vi "Thread Loop.vi"(8 "error in (no error)":errorcluster, 11 "Thread in":refnum<class "Thread.lvclass">) -> (0 "error out":errorcluster, 3 "Thread out":refnum<class "Thread.lvclass">)   [LabVIEW 2012, in "Architecture.lvlib" / "Thread.lvclass"]
uses:
  Thread.lvclass
  Message/Message.lvclass
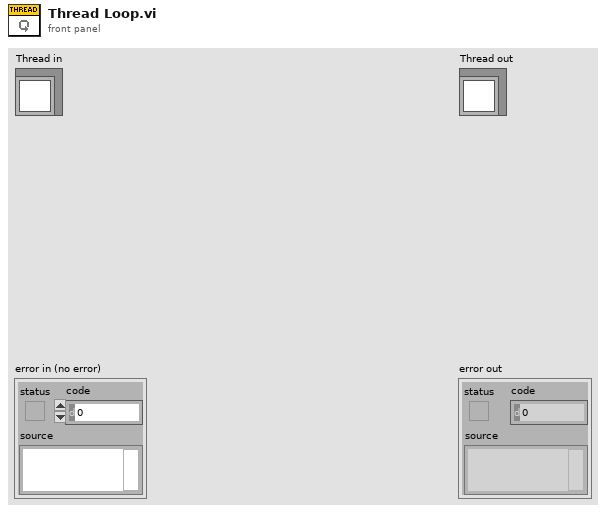
[diagram p1: front panel]
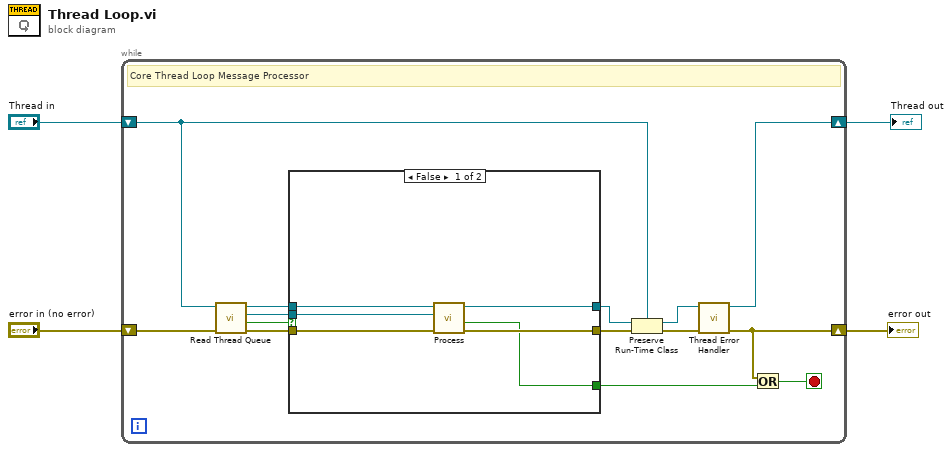
[diagram p0: block diagram]
diagram:
  n1 = while {
    shift-right: [w9] -> w1
    shift-left: "Thread in" -> [w13]
    shift-right: [w7] -> w2
    shift-left: "error in (no error)" -> [w18]
    stop <- w6 stop-if-true
    # "Core Thread Loop Message Processor"
    n2 = call "Read Thread Queue.vi"("error in (no error)"=w18, "Thread in"=w13) -> ("error out"=w16:errorcluster, "timed out?"=w17:bool, "Message"=w8:refnum<class "Message.lvclass">, "Thread out"=w15:refnum<class "Thread.lvclass">)  [unwired: 6 in]
    n3 = case shown="False" w17 {
      tunnel: w16 -> [w24 w25]
      tunnel: [w23 w25] -> w14
      tunnel: w15 -> [w22 w26]
      tunnel: [w21 w26] -> w12
      tunnel: w8 -> [w20 _]
      tunnel: [w19 _] -> w5
      frame False {
        n4 = call-dynamic "Process.vi"("error in (no error)"=w24, "Message in"=w20, "Architecture.lvlib:Thread.lvclass"=w22) -> ("error out"=w23:errorcluster, "Stop?"=w19:bool, "Architecture.lvlib:Thread.lvclass 2"=w21:refnum<class "Thread.lvclass">)  [unwired: 6 in]
      }
      frame True {
      }
    }
    n5 = Preserve Run-Time Class(object in=w12, error in=w14, 2:w13) -> (object out=w11:refnum<class "Thread.lvclass">, error out=w10:errorcluster)
    n6 = call-dynamic "Thread Error Handler.vi"("error in (no error)"=w10, "Thread in"=w11) -> ("error out"=w7:errorcluster, "Thread out"=w9:refnum<class "Thread.lvclass">)  [unwired: 8 in]
    n7 = Or(x=w7, y=w5) -> (x .or. y?=w6:bool)
  }
  "error out" <- w2
  "Thread out" <- w1
